vi "Process Calibration Spreadsheet (TSV).vi"(8 "error in":errorcluster, 11 "Calibration File":path) -> (0 "error out":errorcluster, 1 "intercept":dbl, 2 "slope":dbl, 3 "X - Strain Amplifier (V)":dbl[](array[numeric]), 5 "Y - Load (lbs)":dbl[](array[numeric]))   [LabVIEW 2020]
doc: "Loads a calibration file, computes the best fit curve for the data (by least square method) and reports the slope & intercept."
uses:
  <vilib>/Analysis/6fits.llb/Curve Fitting Criteria.ctl
  <vilib>/Utility/file.llb/Read Delimited Spreadsheet (DBL).vi
  <vilib>/Analysis/NI_AALPro.lvlib
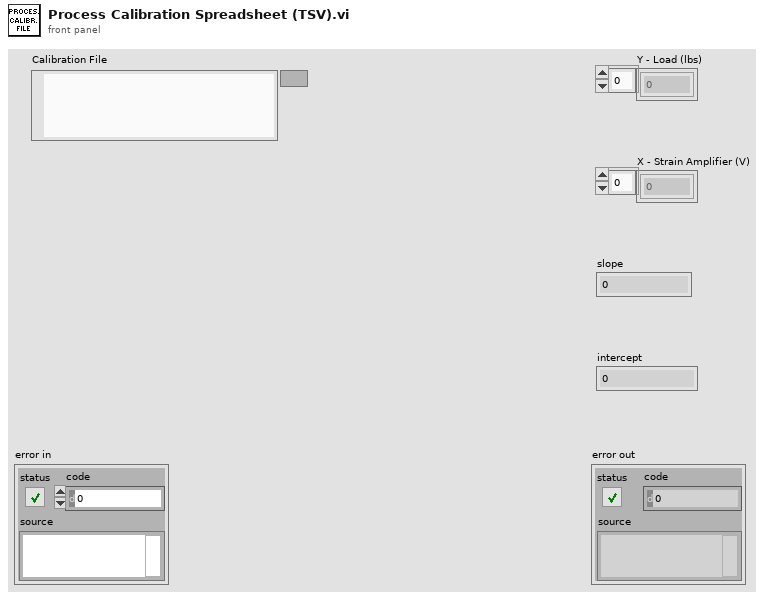
[diagram p1: front panel]
types:
  T1 = typedef "NI_AALPro.lvlib/Curve Fitting Criteria.ctl" = u16
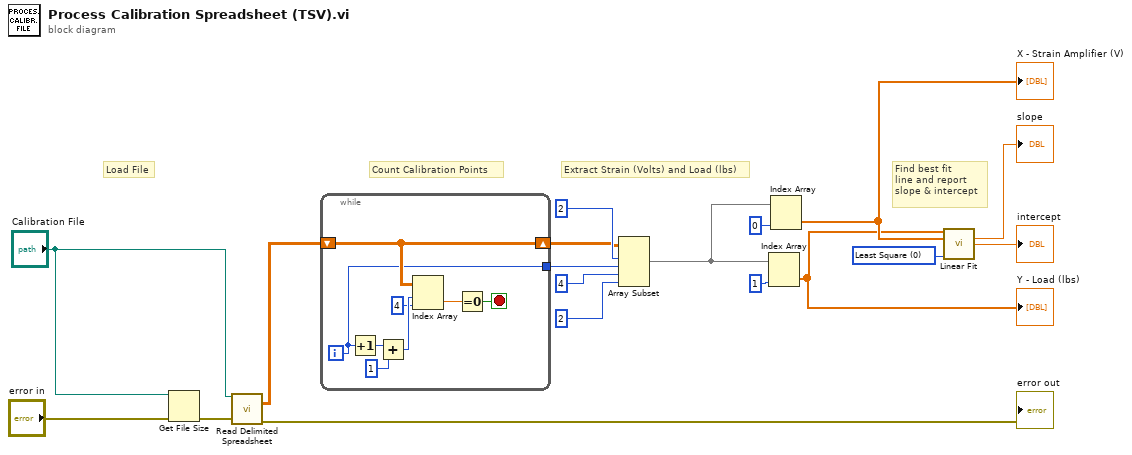
[diagram p0: block diagram]
diagram:
  w15 = T1 0 items=["Least Square", "Least Absolute Residual", "Bisquare"] ("method")
  # "Find best fit\nline and report\nslope & intercept"
  # "Extract Strain (Volts) and Load (lbs)"
  # "Load File"
  # "Count Calibration Points"
  n1 = Get File Size(file="Calibration File", error in="error in") -> (0:w3:errorcluster)  [unwired: 2 out]
  n2 = call-poly <vilib>:"Read Delimited Spreadsheet.vi"("file path (dialog if empty)"="Calibration File", "error in (no error)"=w3) -> ("all rows"=w7:dbl[][], "error out"=→"error out":errorcluster)  [unwired: 8 in, 4 out]
  n3 = while {
    shift-right: [w25] -> w6
    shift-left: w7 -> [w25]
    tunnel: [w19] -> w5
    i -> [w19]
    stop <- w21 stop-if-true
    n4 = Increment(x=w19) -> (x+1=w20:i32)
    n5 = Add(x=w20, y=1) -> (x+y=w23:i32)
    n6 = Index Array(array=w25, index (row)=w23, index (col)=4 ("disabled index (col)")) -> (element=w26:dbl)
    n7 = Equal To 0?(x=w26) -> (x = 0?=w21:bool)
  }
  n8 = Array Subset(array=w6, index (row)=2 ("index"), length (row)=w5, index (col)=4 ("index"), length (col)=2 ("length")) -> (w16:dbl[][])
  n9 = Index Array(array=w16, index (col)=1 ("index (row)")) -> (element=w8:dbl[])  [unwired: 1 in]
  "Y - Load (lbs)" <- w8
  n10 = Index Array(array=w16, index (col)=0 ("index (row)")) -> (element=w9:dbl[])  [unwired: 1 in]
  "X - Strain Amplifier (V)" <- w9
  n11 = call <vilib>:"Linear Fit.vi"("Y"=w8, "X"=w9, "method"=w15) -> ("slope"=→"slope":dbl, "intercept"=→"intercept":dbl)  [unwired: 8 in, 3 out]
